vi "Keithley_BurstRead.vi"() -> ()   [LabVIEW 2015]
panel:
  out "data":string
  in  "Status":i32
  in  "Unit":i32
  in  "Reading number":i32
  in  "Elements to read":i32
  in  "address string":string
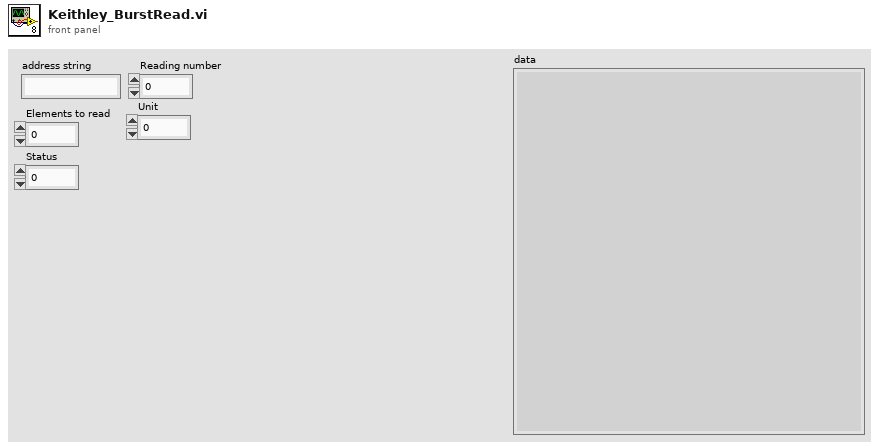
[diagram p1: front panel]
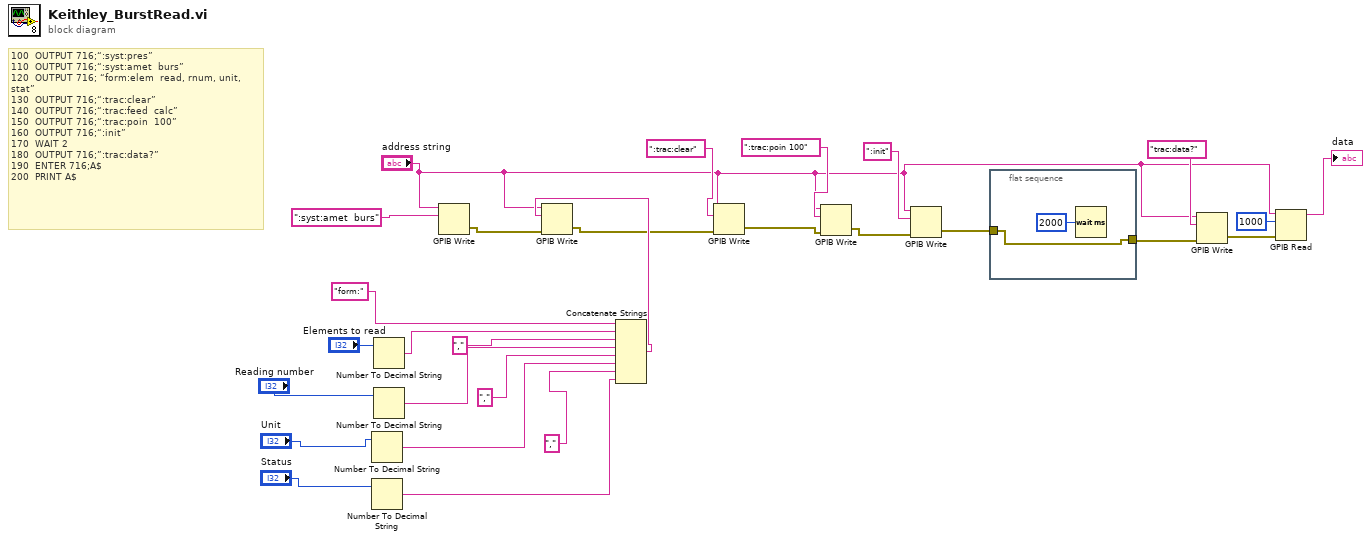
[diagram p0: block diagram]
diagram:
  # "100  OUTPUT 716;“:syst:pres”\n110  OUTPUT 716;“:syst:amet  burs”\n120  OUTPUT 716; “form:elem  read, rnum, unit,\nstat”\n130  OUTPUT 716;“:trac:clear”\n140  OUTPUT 716;“:trac:feed  calc”\n150  OUTPUT 716;“:trac:poin  100”\n160  OUTPUT 716;“:init”\n170  WAIT 2\n180  OUTPUT 716;”:trac:data?”\n190  ENTER 716;A$\n200  PRINT A$"
  n1 = Number To Decimal String(number="Unit") -> (decimal integer string=w20:string)  [unwired: 1 in]
  n2 = Number To Decimal String(number="Status") -> (decimal integer string=w17:string)  [unwired: 1 in]
  n3 = Number To Decimal String(number="Elements to read") -> (decimal integer string=w26:string)  [unwired: 1 in]
  n4 = Number To Decimal String(number="Reading number") -> (decimal integer string=w23:string)  [unwired: 1 in]
  n5 = GPIB Write(0:"address string", 1:":syst:amet  burs" ("data")) -> (6:w15:errorcluster)  [unwired: 3 in, 1 out]
  n6 = Concatenate Strings("form:" ("data"), w26, "," ("string"), w23, "," ("string"), w20, "," ("string"), w17) -> (w14:string)
  n7 = GPIB Write(0:"address string", 1:w14, 3:w15) -> (6:w13:errorcluster)  [unwired: 2 in, 1 out]
  n8 = GPIB Write(0:"address string", 1:":trac:clear" ("data"), 3:w13) -> (6:w11:errorcluster)  [unwired: 2 in, 1 out]
  n9 = GPIB Write(0:"address string", 1:":trac:poin 100" ("data"), 3:w11) -> (6:w9:errorcluster)  [unwired: 2 in, 1 out]
  n10 = GPIB Write(0:"address string", 1:":init" ("data"), 3:w9) -> (6:w7:errorcluster)  [unwired: 2 in, 1 out]
  n11 = flat-sequence {
    tunnel: w7 -> [w29]
    tunnel: [w29] -> w6
    frame #0 {
      n12 = Wait (ms)(milliseconds to wait=u32 2000) -> ()  [unwired: 1 out]
    }
  }
  n13 = GPIB Write(0:"address string", 1:"trac:data?" ("data"), 3:w6) -> (6:w4:errorcluster)  [unwired: 2 in, 1 out]
  n14 = GPIB Read(0:"address string", 1:1000 ("byte count"), 3:w4) -> (5:→"data":string)  [unwired: 2 in, 2 out]
